vi "EOL CAN_Download CAL.vi"(0 "DSC Write Session in":refnum<k21>, 1 "Tester":refnum<k21>, 3 "Download CAL Time":refnum<vi>, 5 "Read Session in":refnum<k21>, 7 "Parttype ref":refnum<vi>, 9 "Glass?":bool=TRUE, 11 "Error String":string, 12 "ODX File Path":path, 14 "Download CAL Progress":refnum<vi>) -> (4 "Response Good?":bool, 6 "TxRx Data":string[][](array[string]), 10 "Error String Out":string, 15 "fail":bool)   [LabVIEW 2014]
uses:
  typedefs/parttype.ctl
panel:
  in  "stop 2":bool
  in  "stop":bool
  out "error out":errorcluster
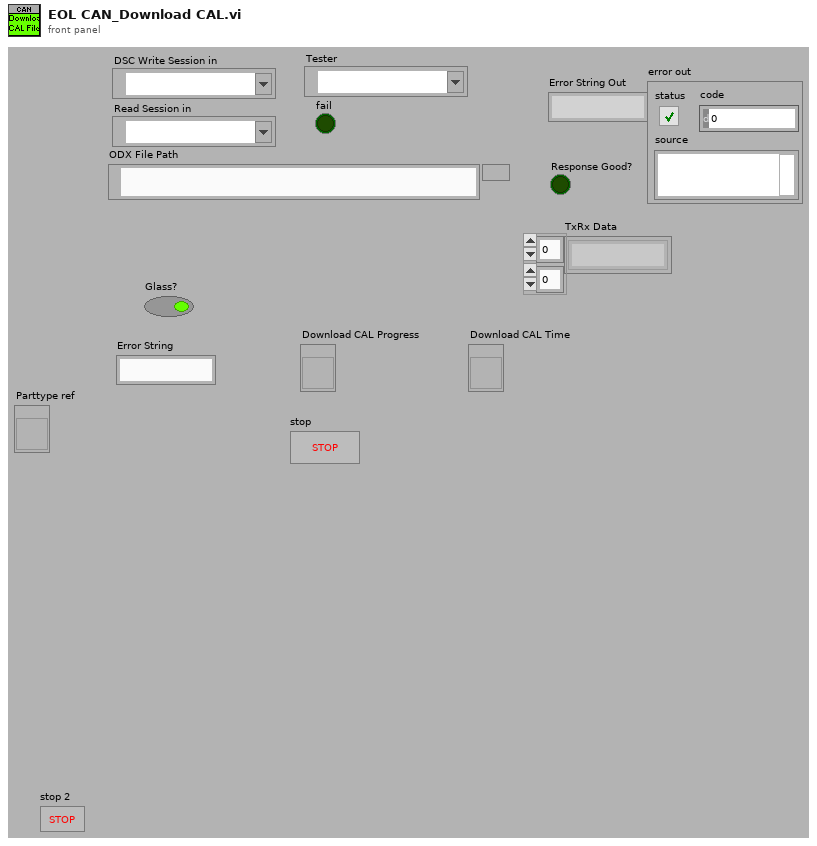
[diagram p1: front panel]
types:
  T1 = cluster{"DSC Write Session in":refnum<k21>, "Read Session in":refnum<k21>, "Error String":string, "Response Good?":bool, "Glass?":bool, "TxRx Data":string[][], "ODX File Path":path, "Flash Data Array":u8[], "Download CAL Progress":refnum<vi>, "Download CAL Time":refnum<vi>, "millisecond timer value":u32, "Parttype ref":refnum<vi>}
  T2 = typedef "Diagnose_SA2_Rechnenbefehl.ctl" = cluster{"Operation":T3, "Wert":u32}
  T3 = typedef "Diagnose_SA2_Operation_ENUM.ctl" = enum16{"RSL", "RSR", "ADD", "SUB", "EOR", "Durchläufe", "NEXT", "BCC", "BRA", "Fertig"}
  T4 = typedef "XNET Frame CAN.ctl" = cluster{"timestamp":timestamp, "payload":u8[], "identifier":u32, "type":T5, "extended?":bool, "echo?":bool}
  T5 = typedef "XNET Frame Type CAN.ctl" = u8
  T6 = cluster{"Start Adress":u8[], "Block Size":u8[], "Checksum":u8[]}
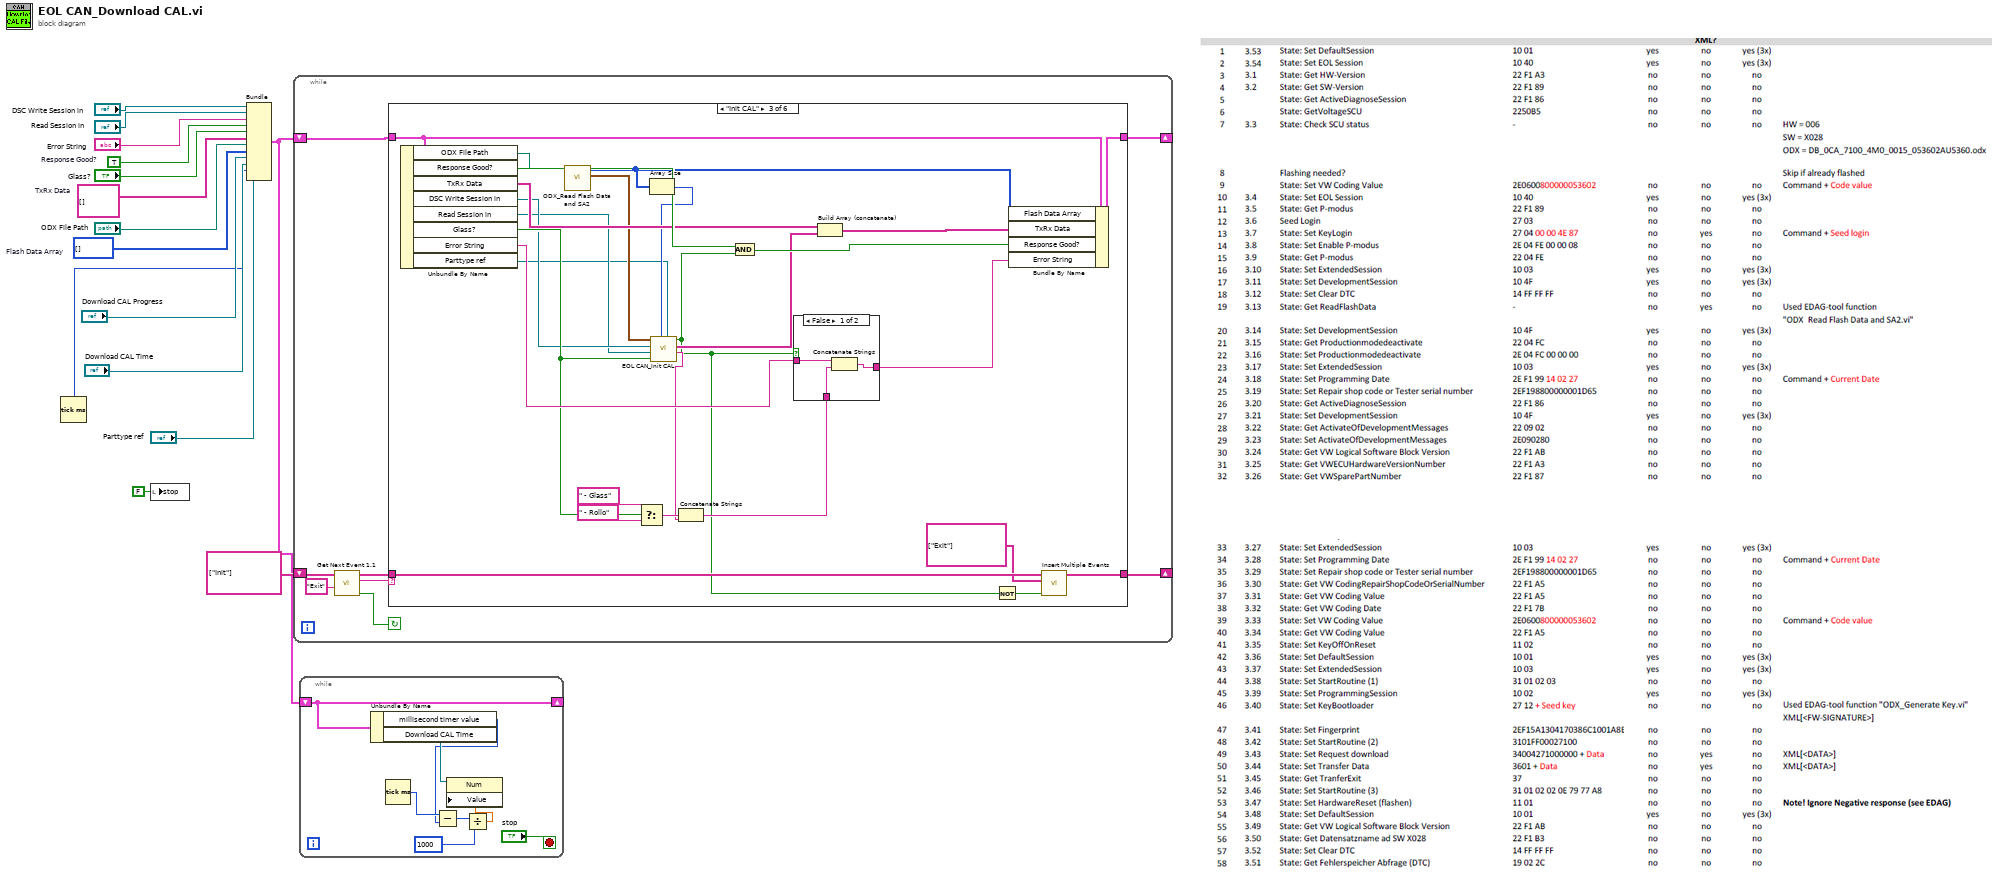
[diagram p0: block diagram]
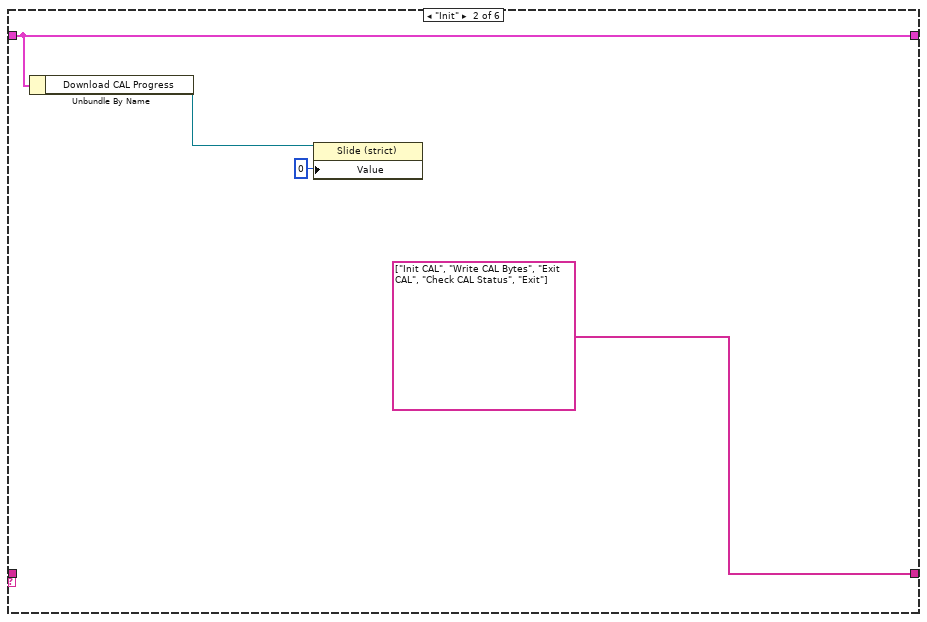
[diagram p3: hidden frame]
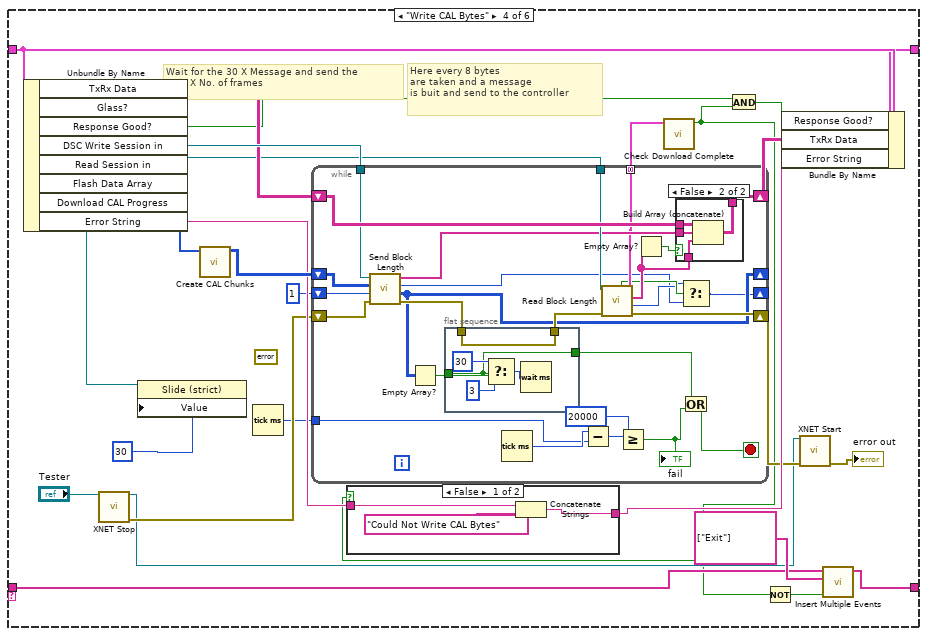
[diagram p5: hidden frame]
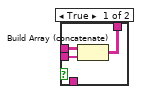
[diagram p6: hidden frame]
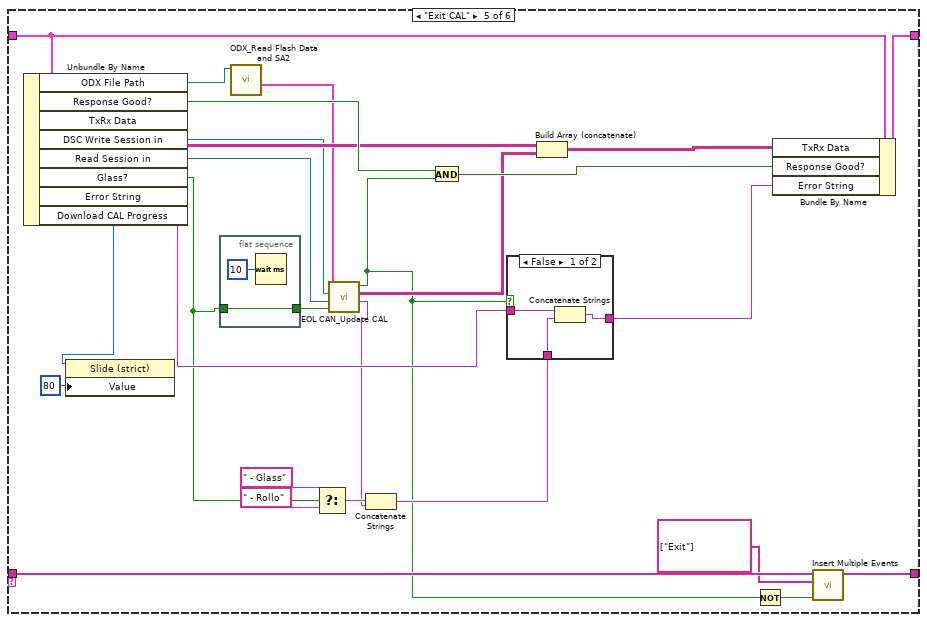
[diagram p8: hidden frame]
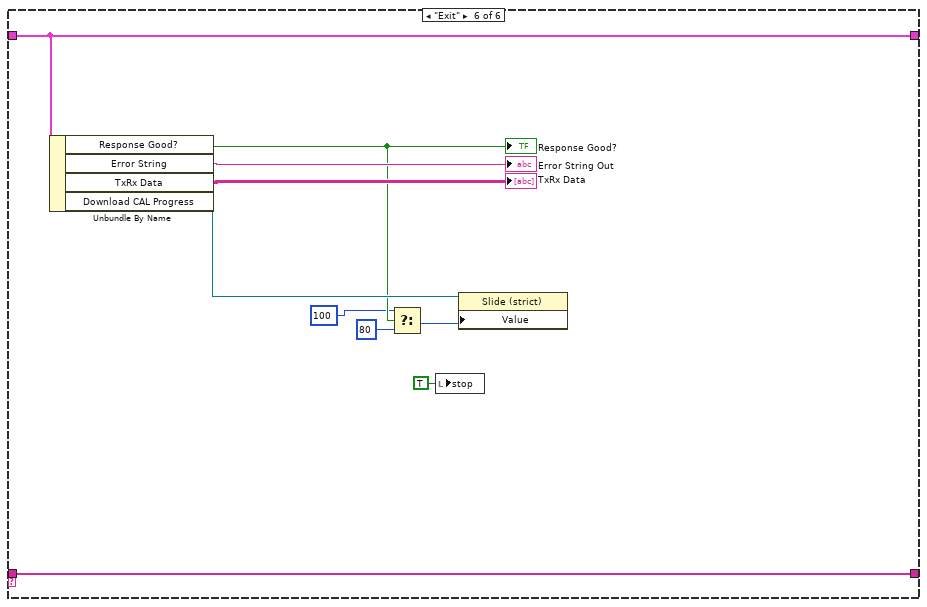
[diagram p10: hidden frame]
diagram:
  w7 = u8[] []  # Flash Data Array
  w11 = string[][] []  # TxRx Data
  w13 = TRUE  # Response Good?
  n1 = Tick Count (ms)() -> (millisecond timer value=w4:u32)
  n2 = local write "stop"(FALSE ("stop")) -> ()
  n3 = Bundle("DSC Write Session in"="DSC Write Session in", "Read Session in"="Read Session in", "Error String"="Error String", "Response Good?"=w13, "Glass?"="Glass?", "TxRx Data"=w11, "ODX File Path"="ODX File Path", "Flash Data Array"=w7, "Download CAL Progress"="Download CAL Progress", "Download CAL Time"="Download CAL Time", "millisecond timer value"=w4, "Parttype ref"="Parttype ref") -> (w3:T1)  [unwired: 1 in]
  n4 = while {
    shift-right: [w21] -> _
    shift-left: string[] ["Init"] ("event queue out") -> [w20]
    shift-right: [w19] -> _
    shift-left: w3 -> [w16]
    stop <- w23 continue-if-true
    n5 = call "Get Next Event 1.1.vi"("Exit Event"="Exit", "event queue in"=w20) -> ("Condition (Exit:F)"=w23:bool, "next event"=w17:string, "event queue out"=w22:string[])  [unwired: 6 in, 1 out]
    n6 = case shown="\"Init CAL\"" w17 {
      tunnel: w22 -> [w25 _ w45 w75 w154 w173]
      tunnel: [w25 string[] ["Init CAL", "Write CAL Bytes", "Exit CAL", "Check CAL Status", "Exit"] ("event queue out") w46 w76 w155 w173] -> w21
      tunnel: w16 -> [w24 w26 w55 w87 w157 w172]
      tunnel: [w24 w26 w53 w86 w156 w172] -> w19
      frame "Error", Default {
      }
      frame "Init" {
        n7 = Unbundle By Name(w26) -> ("Download CAL Progress"=w28:refnum<vi>)
        n8 = property class="Slide (strict)"(reference=w28, "Value"=u8 0) -> ()  [unwired: 1 in, 2 out]
      }
      frame "Init CAL" {
        n9 = Unbundle By Name(w55) -> ("ODX File Path"=w40:path, "Response Good?"=w56:bool, "TxRx Data"=w43:string[][], "DSC Write Session in"=w34:refnum<k21>, "Read Session in"=w33:refnum<k21>, "Glass?"=w35:bool, "Error String"=w52:string, "Parttype ref"=w30:refnum<vi>)
        n10 = call "ODX_Read Flash Data and SA2.vi"("ODX File Path"=w40) -> ("SA2 Operator"=w41:T2[], "Flash Data Array"=w32:u8[])  [unwired: 7 in, 2 out]
        n11 = Select(t=" - Glass" ("Error Description"), s=w35, f=" - Rollo" ("Error Description")) -> (s? t:f=w50:string)
        n12 = Array Size(array=w32) -> (size(s)=w31:i32)
        n13 = call "EOL CAN_Init CAL.vi"("Parttype ref"=w30, "Flash Size"=w31, "Glass?"=w35, "Read Session in"=w33, "DSC Write Session in"=w34, "SA2 Operator"=w41) -> ("Error String Out"=w38:string, "TxRx Data"=w39:string[][], "Response Good?"=w37:bool)  [unwired: 3 in]
        n14 = Concatenate Strings(w50, w38) -> (w47:string)
        n15 = And(x=w56, y=w37) -> (x .and. y?=w54:bool)
        n16 = case shown="False" w37 {
          tunnel: w52 -> [w58 w60]
          tunnel: [w59 w60] -> w51
          tunnel: w47 -> [w57 _]
          frame False {
            n17 = Concatenate Strings(w58, w57) -> (w59:string)
          }
          frame True {
          }
        }
        n18 = Build Array (concatenate)(w43, w39) -> (w42:string[][])
        n19 = Not(x=w37) -> (.not. x?=w36:bool)
        n20 = Bundle By Name(cluster=w55, "Flash Data Array"=w32, "TxRx Data"=w42, "Response Good?"=w54, "Error String"=w51) -> (w53:T1)
        n21 = call "Insert Multiple Events.vi"("Insert all? (T)"=w36, "Events to Insert"=string[] ["Exit"], "Event queue in"=w45) -> ("Event queue out"=w46:string[])  [unwired: 4 in]
      }
      frame "Write CAL Bytes" {
        (unwired) errorcluster {"status"=FALSE, "code"=0, "source"=""} ("error out 2")
        # "Wait for the 30 X Message and send the\nnext X No. of frames"
        # "Here every 8 bytes\nare taken and a message\nis buit and send to the controller"
        n22 = Unbundle By Name(w87) -> ("TxRx Data"=w84:string[][], "Response Good?"=w80:bool, "DSC Write Session in"=w85:refnum<k21>, "Read Session in"=w79:refnum<k21>, "Flash Data Array"=w62:u8[], "Download CAL Progress"=w73:refnum<vi>, "Error String"=w72:string)  [unwired: 1 out]
        n23 = call <vilib>:"XNET Stop.vi"("session in"="Tester") -> ("session out"=w67:refnum<k21>, "error out"=w69:errorcluster)  [unwired: 13 in]
        n24 = property class="Slide (strict)"(reference=w73, "Value"=u8 30) -> ()  [unwired: 1 in, 2 out]
        n25 = call "Create CAL Chunks.vi"("Flash Data Array"=w62) -> ("Array 2"=w83:u8[][])  [unwired: 10 in]
        n26 = Tick Count (ms)() -> (millisecond timer value=w61:u32)
        n27 = while {
          tunnel: w85 -> [w112]
          shift-right: [w113] -> w82
          shift-left: w84 -> [w114]
          tunnel: w79 -> [w111]
          tunnel: [w109] -> w65 mode=concatenating
          shift-right: [w104] -> w68
          shift-left: w69 -> [w103]
          shift-right: [w95] -> _
          shift-left: u16 1 ("Block Size") -> [w102]
          shift-right: [w98] -> _
          shift-left: w83 -> [w100]
          tunnel: w61 -> [w92]
          stop <- w89 stop-if-true
          n28 = call "Send Block Length.vi"("error in (no error)"=w103, "Block Size In"=w102, "Array in"=w100, "Refnum in"=w112) -> ("error out"=w106:errorcluster, "Array Out"=w98:u8[][], "Block Size Out"=w94:u32, "Array out"=w110:string[])  [unwired: 4 in]
          n29 = Empty Array?(array=w98) -> (empty?=w101:bool)
          n30 = flat-sequence {
            tunnel: w106 -> [w119]
            tunnel: [w119] -> w105
            tunnel: w101 -> [w115]
            tunnel: [w115] -> w99
            frame #0 {
              n31 = Select(t=u32 30, s=w115, f=u32 3 ("milliseconds to wait")) -> (s? t:f=w118:u32)
              n32 = Wait (ms)(milliseconds to wait=w118) -> ()  [unwired: 1 out]
            }
          }
          n33 = Tick Count (ms)() -> (millisecond timer value=w93:u32)
          n34 = Subtract(x=w93, y=w92) -> (x-y=w91:u32)
          n35 = call "Read Block Length.vi"("error in (no error)"=w105, "Refnum in"=w111) -> ("error out"=w104:errorcluster, "Block Size"=w96:u16, "Array"=w107:string[], "data"=w109:T4[], "Flow Control?"=w97:bool)  [unwired: 5 in]
          n36 = Greater Or Equal?(x=w91, y=u32 20000) -> (x >= y?=w88:bool)
          "fail" <- w88
          n37 = Empty Array?(array=w107) -> (empty?=w108:bool)
          n38 = case shown="False" w108 {
            tunnel: w114 -> [w122 w126]
            tunnel: [w121 w125] -> w113
            tunnel: w110 -> [w120 w124]
            tunnel: w107 -> [_ w123]
            frame True {
              n39 = Build Array (concatenate)(w122, w120) -> (w121:string[][])
            }
            frame False {
              n40 = Build Array (concatenate)(w126, w124, w123) -> (w125:string[][])
            }
          }
          n41 = Select(t=w96, s=w97, f=w94) -> (s? t:f=w95:u32)
          n42 = Or(x=w99, y=w88) -> (x .or. y?=w89:bool)
        }
        n43 = call "Check Download Complete.vi"("data"=w65) -> ("Boolean"=w64:bool)  [unwired: 10 in]
        n44 = case shown="False" w64 {
          tunnel: w72 -> [w129 w130]
          tunnel: [w127 w130] -> w71
          frame False {
            n45 = Concatenate Strings(w129, "Could Not Write CAL Bytes" ("string")) -> (w127:string)
          }
          frame True {
          }
        }
        n46 = And(x=w80, y=w64) -> (x .and. y?=w81:bool)
        n47 = Not(x=w64) -> (.not. x?=w77:bool)
        n48 = Bundle By Name(cluster=w87, "Response Good?"=w81, "TxRx Data"=w82, "Error String"=w71) -> (w86:T1)
        n49 = call <vilib>:"XNET Start.vi"("session in"=w67, "error in (no error)"=w68) -> ("error out"=→"error out":errorcluster)  [unwired: 12 in, 1 out]
        n50 = call "Insert Multiple Events.vi"("Insert all? (T)"=w77, "Events to Insert"=string[] ["Exit"], "Event queue in"=w75) -> ("Event queue out"=w76:string[])  [unwired: 4 in]
      }
      frame "Exit CAL" {
        n51 = Unbundle By Name(w157) -> ("ODX File Path"=w136:path, "Response Good?"=w153:bool, "TxRx Data"=w144:string[][], "DSC Write Session in"=w141:refnum<k21>, "Read Session in"=w140:refnum<k21>, "Glass?"=w134:bool, "Error String"=w151:string, "Download CAL Progress"=w131:refnum<vi>)
        n52 = property class="Slide (strict)"(reference=w131, "Value"=u8 80) -> ()  [unwired: 1 in, 2 out]
        n53 = flat-sequence {
          tunnel: w134 -> [w158]
          tunnel: [w158] -> w133
          frame #0 {
            n54 = Wait (ms)(milliseconds to wait=u32 10) -> ()  [unwired: 1 out]
          }
        }
        n55 = call "ODX_Read Flash Data and SA2.vi"("ODX File Path"=w136) -> ("Download Parameter"=w135:T6)  [unwired: 7 in, 3 out]
        n56 = Select(t=" - Glass" ("Error Description"), s=w134, f=" - Rollo" ("Error Description")) -> (s? t:f=w149:string)
        n57 = call "EOL CAN_Update CAL.vi"("Glass?"=w133, "Read Session in"=w140, "DSC Write Session in"=w141, "Download Parameter"=w135) -> ("Error String Out"=w138:string, "TxRx Data"=w139:string[][], "Response Good?"=w137:bool)  [unwired: 5 in]
        n58 = Concatenate Strings(w149, w138) -> (w146:string)
        n59 = And(x=w153, y=w137) -> (x .and. y?=w152:bool)
        n60 = case shown="False" w137 {
          tunnel: w151 -> [w161 w163]
          tunnel: [w162 w163] -> w150
          tunnel: w146 -> [w160 _]
          frame False {
            n61 = Concatenate Strings(w161, w160) -> (w162:string)
          }
          frame True {
          }
        }
        n62 = Build Array (concatenate)(w144, w139) -> (w143:string[][])
        n63 = Not(x=w137) -> (.not. x?=w142:bool)
        n64 = Bundle By Name(cluster=w157, "TxRx Data"=w143, "Response Good?"=w152, "Error String"=w150) -> (w156:T1)
        n65 = call "Insert Multiple Events.vi"("Insert all? (T)"=w142, "Events to Insert"=string[] ["Exit"], "Event queue in"=w154) -> ("Event queue out"=w155:string[])  [unwired: 4 in]
      }
      frame "Exit" {
        n66 = Unbundle By Name(w172) -> ("Response Good?"=w167:bool, "Error String"=→"Error String Out":string, "TxRx Data"=→"TxRx Data":string[][], "Download CAL Progress"=w169:refnum<vi>)
        "Response Good?" <- w167
        n67 = Select(t=u8 100 ("Value"), s=w167, f=u8 80) -> (s? t:f=w164:u8)
        n68 = local write "stop"(TRUE ("stop")) -> ()
        n69 = property class="Slide (strict)"(reference=w169, "Value"=w164) -> ()  [unwired: 1 in, 2 out]
      }
    }
  }
  n70 = while {
    shift-right: [w176] -> _
    shift-left: w3 -> [w176]
    stop <- "stop" stop-if-true
    n71 = Unbundle By Name(w176) -> ("millisecond timer value"=w175:u32, "Download CAL Time"=w180:refnum<vi>)
    n72 = Tick Count (ms)() -> (millisecond timer value=w177:u32)
    n73 = Subtract(x=w177, y=w175) -> (x-y=w178:u32)
    n74 = Divide(x=w178, y=u32 1000) -> (x/y=w181:dbl)
    n75 = property class="Num"(reference=w180, "Value"=w181) -> ()  [unwired: 1 in, 2 out]
  }
